vi "OngoingBumpsToggled.vi"(6 "Override bumps":bool, 7 "DO Task":refnum<k21>="BlueSimple_DO", 8 "Start \nbump timer?":bool, 9 "Bump Parameters":T1={"Distance (deg)"=2.0, "Travel time (ms)"=500.0} {"Travel time (ms)" min=0.1 max=10000.0; "Distance (deg)" min=0.1}, 10 "Bump timing":cluster{"Fix":dbl, "Rnd":dbl}={"Fix"=0.5, "Rnd"=0.5} {"Rnd" format="%.4f"; "Fix" format="%_4g"}, 11 "Bumps on?":bool) -> (0 "Reset start button":bool, 1 "Reset override bumps":bool)   [LabVIEW 2010]
panel:
  # "+"
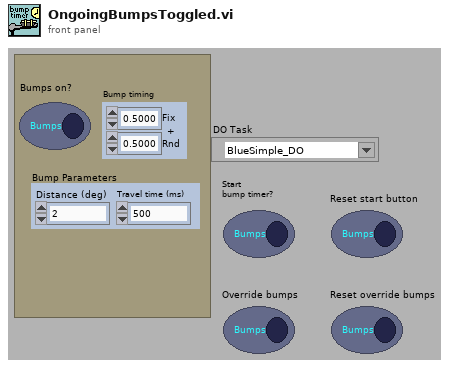
[diagram p1: front panel]
types:
  T1 = cluster{"Distance (deg)":dbl, "Travel time (ms)":dbl}
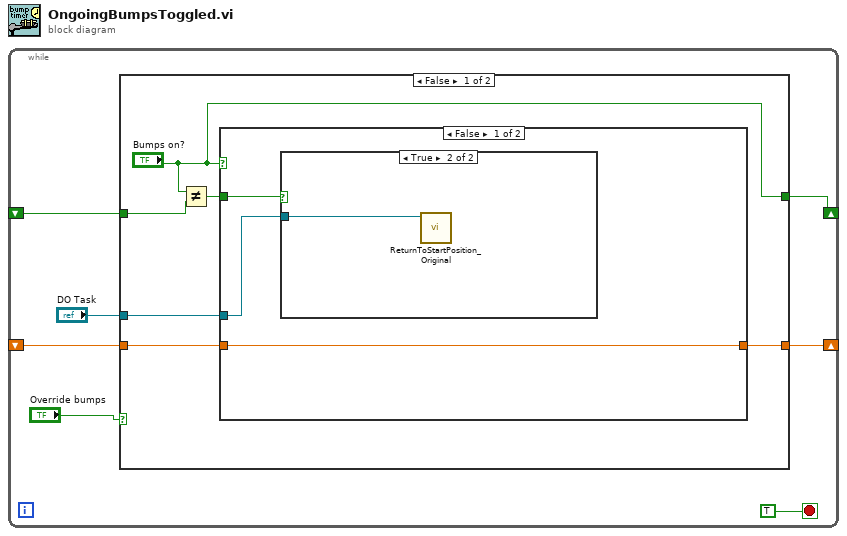
[diagram p0: block diagram]
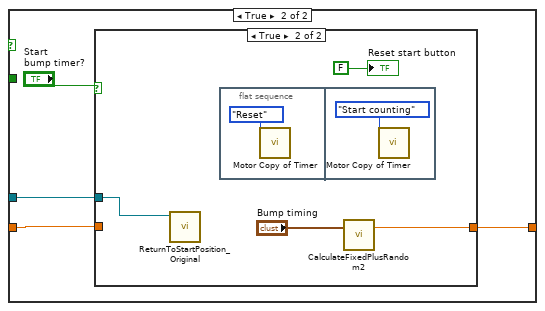
[diagram p3: hidden frame]
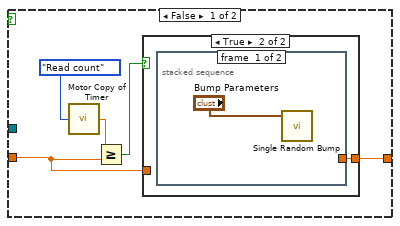
[diagram p4: hidden frame]
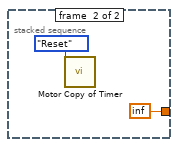
[diagram p6: hidden frame]
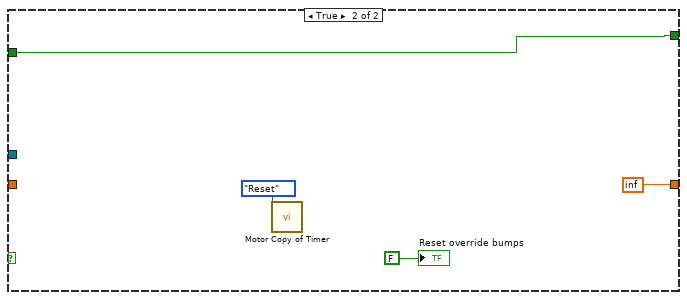
[diagram p7: hidden frame]
diagram:
  n1 = while {
    shift-right: [w7] -> _
    shift-left: _ -> [w6]
    shift-right: [w4] -> _
    shift-left: _ -> [w5]
    stop <- TRUE stop-if-true
    n2 = case shown="False" "Override bumps" {
      tunnel: [w13 inf] -> w7
      tunnel: w6 -> [w12 _]
      tunnel: w5 -> [w11 w38]
      tunnel: ["Bumps on?" w38] -> w4
      tunnel: "DO Task" -> [w8 _]
      frame False {
        n3 = Not Equal?(x="Bumps on?", y=w11) -> (x != y?=w10:bool)
        n4 = case shown="False" "Bumps on?" {
          tunnel: [w16 w21] -> w13
          tunnel: w12 -> [w16 w20]
          tunnel: w10 -> [w15 _]
          tunnel: w8 -> [w14 w18]
          frame False {
            n5 = case shown="True" w15 {
              tunnel: w14 -> [_ w17]
              frame False {
              }
              frame True {
                n6 = call "ReturnToStartPosition_Original.vi"("DO Task"=w17) -> ()  [unwired: 9 in]
              }
            }
          }
          frame True {
            n7 = case shown="True" "Start \nbump timer?" {
              tunnel: [w23 w35] -> w21
              tunnel: w20 -> [w22 _]
              tunnel: w18 -> [_ w32]
              frame False {
                n8 = call "Motor Copy of Timer.vi"("Command"=enum16{"Start counting", "Read count", "Reset"}."Read count") -> ("Time out"=w25:dbl)
                n9 = Greater Or Equal?(x=w25, y=w22) -> (x >= y?=w26:bool)
                n10 = case shown="True" w26 {
                  tunnel: [w27 w28] -> w23
                  tunnel: w22 -> [w27 _]
                  frame False {
                  }
                  frame True {
                    n11 = stacked-sequence {
                      tunnel: [_ inf] -> w28
                      frame #0 {
                        n12 = call "Single Random Bump.vi"("Bump Parameters"="Bump Parameters") -> ()  [unwired: 7 in]
                      }
                      frame #1 {
                        n13 = call "Motor Copy of Timer.vi"("Command"=enum16{"Start counting", "Read count", "Reset"}."Reset") -> ()  [unwired: 1 out]
                      }
                    }
                  }
                }
              }
              frame True {
                n14 = call "ReturnToStartPosition_Original.vi"("DO Task"=w32) -> ()  [unwired: 9 in]
                n15 = flat-sequence {
                  frame #0 {
                    n16 = call "Motor Copy of Timer.vi"("Command"=enum16{"Start counting", "Read count", "Reset"}."Reset") -> ()  [unwired: 1 out]
                  }
                  frame #1 {
                    n17 = call "Motor Copy of Timer.vi"("Command"=enum16{"Start counting", "Read count", "Reset"}."Start counting") -> ()  [unwired: 1 out]
                  }
                }
                n18 = call "CalculateFixedPlusRandom2.vi"("Component times"="Bump timing") -> ("Composite time"=w35:dbl)  [unwired: 1 in, 1 out]
                "Reset start button" <- FALSE ("Reset start button")
              }
            }
          }
        }
      }
      frame True {
        n19 = call "Motor Copy of Timer.vi"("Command"=enum16{"Start counting", "Read count", "Reset"}."Reset") -> ()  [unwired: 1 out]
        "Reset override bumps" <- FALSE ("Reset override bumps")
      }
    }
  }
